vi "tajmer.vi"(8 "error in (no error)":errorcluster, 9 "ulazni podaci tajmera":T2, 10 "Vrijeme od kog se broji":dbl, 11 "Enum":T3) -> (0 "error out":errorcluster, 1 "izlazni podaci tajmera":T2, 3 "status tajmera":T1)   [LabVIEW 2023]
uses:
  tajmer_kontrola.ctl
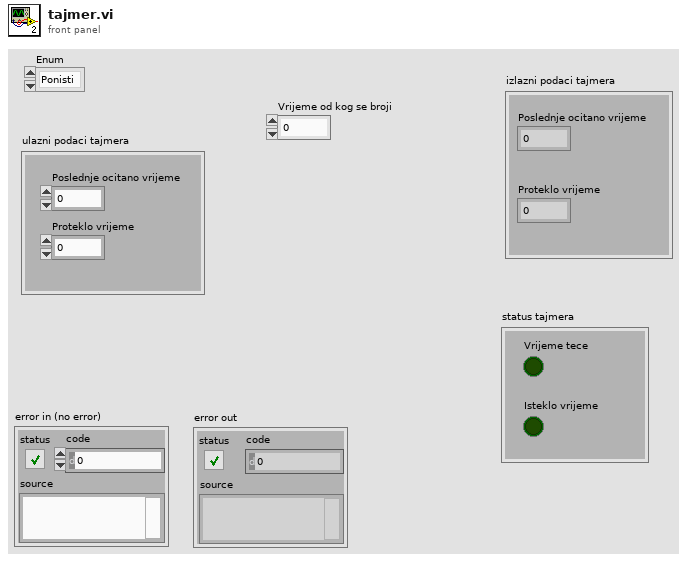
[diagram p1: front panel]
types:
  T1 = cluster{"Vrijeme tece":bool, "Isteklo vrijeme":bool}
  T2 = cluster{"Poslednje ocitano vrijeme":dbl, "Proteklo vrijeme":dbl}
  T3 = typedef "tajmer_kontrola.ctl" = enum16{"Ponisti", "Provjeri"}
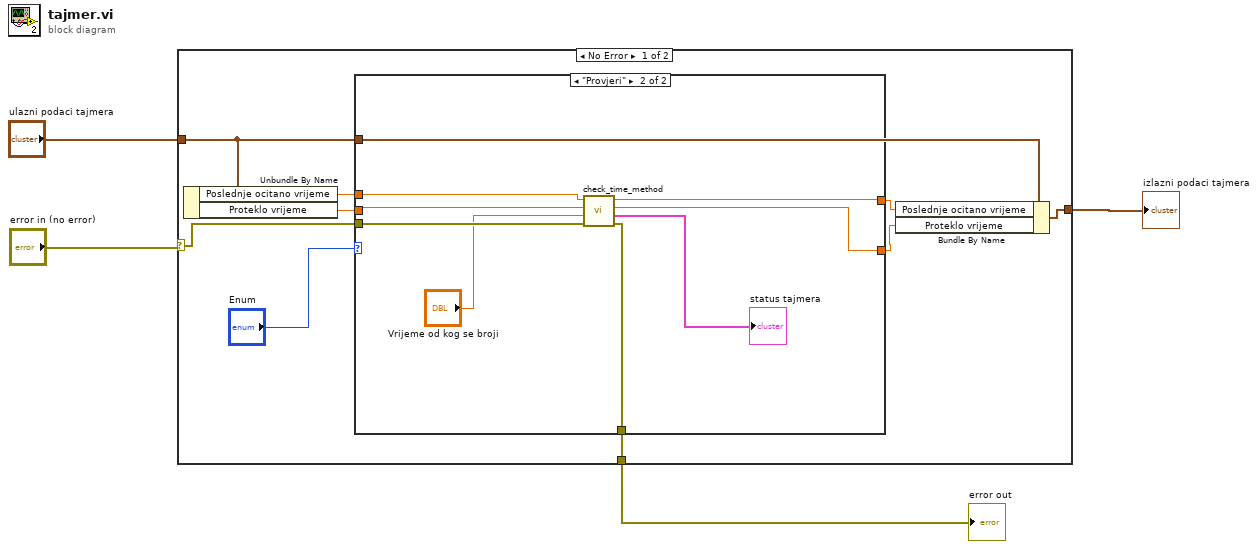
[diagram p0: block diagram]
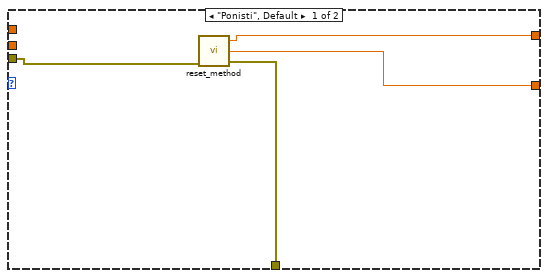
[diagram p2: hidden frame]
diagram:
  n1 = case shown="No Error" "error in (no error)" {
    selector: "error in (no error)" -> [w10 w27]
    tunnel: "ulazni podaci tajmera" -> [w8 w26]
    tunnel: [w9 w27] -> w2
    tunnel: [w7 w26] -> w1
    frame No Error {
      n2 = Unbundle By Name(w8) -> ("Poslednje ocitano vrijeme"=w12:dbl, "Proteklo vrijeme"=w11:dbl)
      n3 = case shown="\"Provjeri\"" "Enum" {
        tunnel: w8 -> [_ _]
        tunnel: w12 -> [_ w25]
        tunnel: w11 -> [_ w24]
        tunnel: w10 -> [w16 w23]
        tunnel: [w17 w20] -> w9
        tunnel: [w15 w19] -> w6
        tunnel: [w14 w18] -> w5
        frame "Ponisti", Default {
          n4 = call "reset_method.vi"("error in (no error)"=w16) -> ("Novo proteklo vrijeme"=w15:dbl, "Novi vremenski trenutak"=w14:dbl, "error out"=w17:errorcluster)  [unwired: 5 in]
        }
        frame "Provjeri" {
          n5 = call "check_time_method.vi"("error in (no error)"=w23, "Vrijeme od kog se broji"="Vrijeme od kog se broji", "Proteklo vrijeme"=w24, "Poslednji vremenski trenutak"=w25) -> ("error out"=w20:errorcluster, "Status"=→"status tajmera":T1, "Novo proteklo vrijeme"=w18:dbl, "Novi vremenski trenutak"=w19:dbl)  [unwired: 4 in]
        }
      }
      n6 = Bundle By Name(cluster=w8, "Poslednje ocitano vrijeme"=w6, "Proteklo vrijeme"=w5) -> (w7:T2)
    }
    frame Error {
    }
  }
  "error out" <- w2
  "izlazni podaci tajmera" <- w1
